vi "LabView_Knob_Multiple_LED.vi"() -> ()   [LabVIEW 2020]
uses:
  <vilib>/Instr/_visa.llb/VISA Configure Serial Port (Instr).vi
panel:
  in  "Tab Control":enum32{"README", "Program"}(tab)
  in  "Folder structure":string(tree)
  in  "GREEN":dbl(knob) scale=0.0..255.0
  in  "BLUE":dbl(knob) scale=0.0..255.0
  in  "stop":bool
  out "Change in value detected":bool
  in  "RED":dbl(knob) scale=0.0..255.0
  in  "Choose VISA resource":refnum<visa-resource-name>
  out "String (passed to Arduino)":string
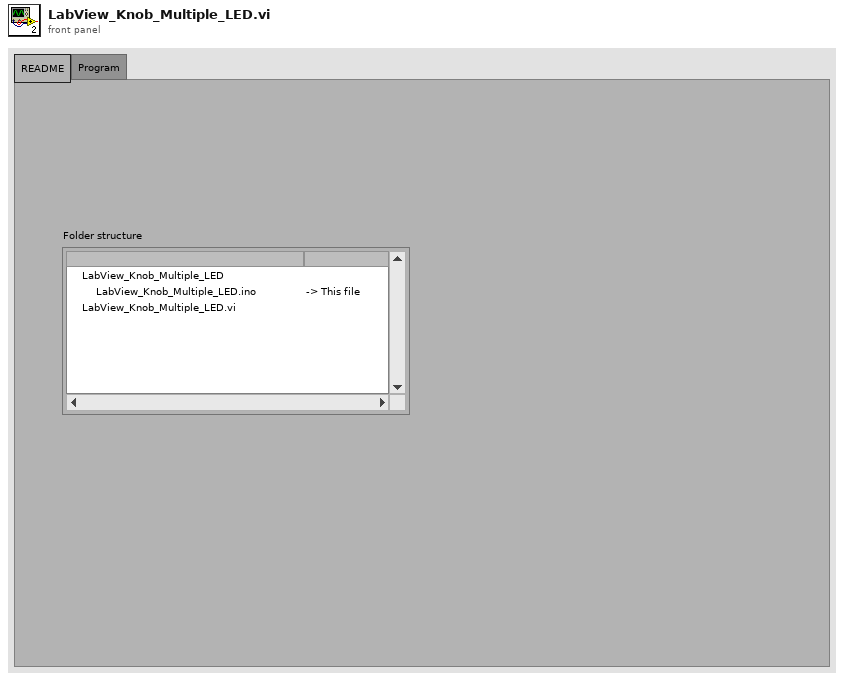
[diagram p1: front panel]
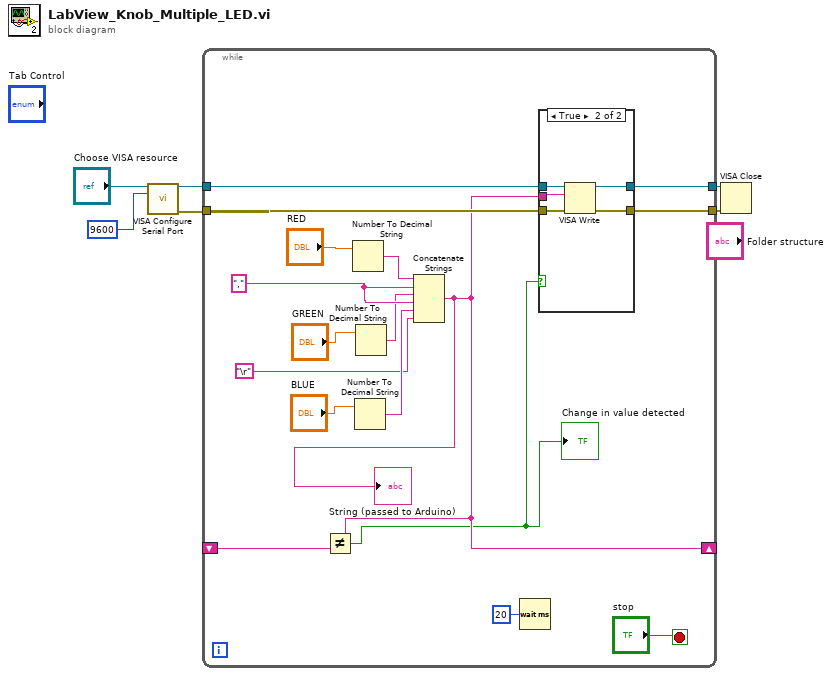
[diagram p0: block diagram]
diagram:
  n1 = call-poly "VISA Configure Serial Port"("VISA resource name"="Choose VISA resource", "baud rate (9600)"=u32 9600) -> ("VISA resource name out"=w2:refnum<visa-resource-name>, "error out"=w1:errorcluster)  [unwired: 12 in]
  n2 = while {
    tunnel: w2 -> [w21]
    tunnel: [w20] -> w5
    tunnel: w1 -> [w19]
    tunnel: [w18] -> w4
    shift-right: [w9] -> _
    shift-left: _ -> [w16]
    stop <- "stop" stop-if-true
    w12 = ","
    n3 = Number To Decimal String(number="RED") -> (decimal integer string=w22:string)  [unwired: 1 in]
    n4 = Number To Decimal String(number="BLUE") -> (decimal integer string=w10:string)  [unwired: 1 in]
    n5 = Number To Decimal String(number="GREEN") -> (decimal integer string=w11:string)  [unwired: 1 in]
    n6 = Concatenate Strings(w22, w12, w11, w12, w10, "\r") -> (w9:string)
    "String (passed to Arduino)" <- w9
    n7 = Not Equal?(x=w9, y=w16) -> (x != y?=w7:bool)
    "Change in value detected" <- w7
    n8 = Wait (ms)(milliseconds to wait=u32 20) -> ()  [unwired: 1 out]
    n9 = case shown="True" w7 {
      tunnel: w21 -> [w25 w30]
      tunnel: [w25 w29] -> w20
      tunnel: w19 -> [w24 w28]
      tunnel: [w24 w27] -> w18
      tunnel: w9 -> [_ w26]
      frame False {
      }
      frame True {
        n10 = VISA Write(VISA resource name=w30, write buffer=w26, error in (no error)=w28) -> (VISA resource name out=w29:refnum<visa-resource-name>, error out=w27:errorcluster)  [unwired: 1 out]
      }
    }
  }
  n11 = VISA Close(VISA resource name=w5, error in (no error)=w4) -> ()  [unwired: 1 out]
